vi "FGV Automatic start.vi"(11 "error in (no error)":errorcluster caption="Fehler (Eingang, kein Fehler)", 13 "Aktion":T1) -> (4 "Starten":bool, 8 "AK Start":bool, 15 "error out":errorcluster caption="Fehler (Ausgang)")   [LabVIEW 2020, in "EPA 1065.lvlib" / "Dichtheitstest 1065-345.lvlib"]
uses:
  Dichtheitstest 1065-345.lvlib
  Aktion FGV Automatic start.ctl
  Bildwechsel/Bild-Auswahl.ctl
  Bildwechsel/Bildwechsel.lvlib
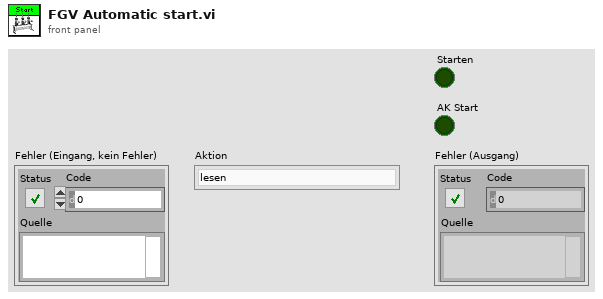
[diagram p1: front panel]
types:
  T1 = typedef "EPA 1065.lvlib/Dichtheitstest 1065-345.lvlib/Aktion FGV Automatic start.ctl" = enum16{"lesen", "Test starten aktiv", "Test starten inaktiv", "Seite merken", "Seite zurücksetzen", "AK Start inaktiv"}
  T2 = typedef "Bildwechsel.lvlib/Bild-Auswahl.ctl" = enum16{"lesen", "Initialisieren", "Beenden", "Grafik", "Anlagenübersicht", "Anlagengrenzwerte", "Log Konfig", "Gaszuordnung AO", "Erw. Konfiguration", "FT-IR  ", "Störmeldungen", "Störmeldepuffer", "Störmeldekonfig", "PNS Grenzwerte", "Statusübersicht", "Linearisierung", "ARN", "EPA Dichtheitstest", "FID", "PMA", "CalGas", "Lambda", "Interference", "Amium PNS", "EPA T90", "Interference N2O", "Scheduler", "Systemeinstellungen", "EPA Drift", "CAN Konfig"}
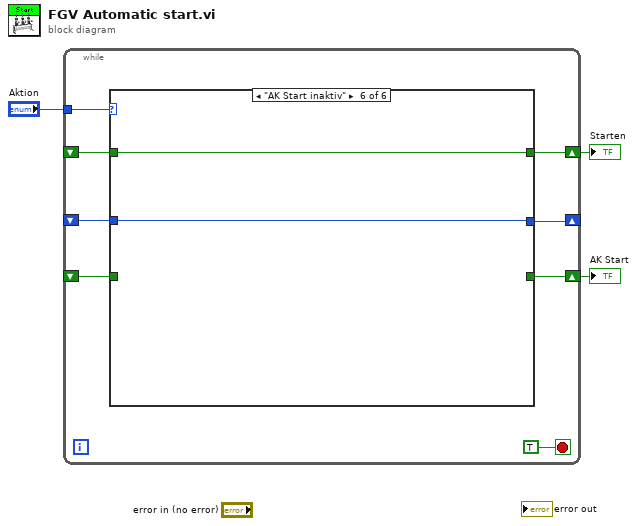
[diagram p0: block diagram]
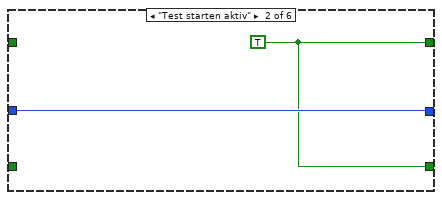
[diagram p3: hidden frame]
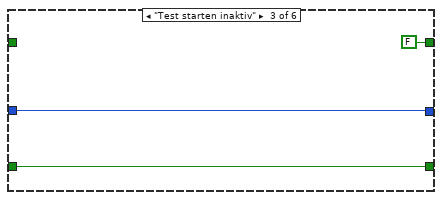
[diagram p4: hidden frame]
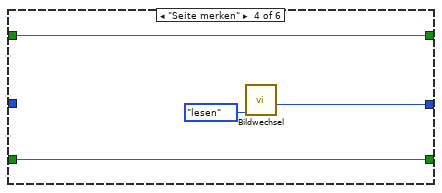
[diagram p5: hidden frame]
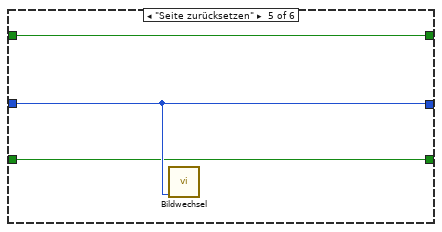
[diagram p6: hidden frame]
diagram:
  n1 = while {
    tunnel: "Aktion" -> [w10]
    shift-right: [w9] -> w2
    shift-left: _ -> [w8]
    shift-right: [w7] -> _
    shift-left: _ -> [w6]
    shift-right: [w5] -> w1
    shift-left: _ -> [w4]
    stop <- TRUE stop-if-true
    n2 = case shown="\"AK Start inaktiv\"" w10 {
      tunnel: [w14 w15 FALSE w23 w26 w27] -> w9
      tunnel: w8 -> [w14 _ _ w23 w26 w27]
      tunnel: [w13 w16 w18 w21 w25 w28] -> w7
      tunnel: w6 -> [w13 w16 w18 _ w25 w28]
      tunnel: [w12 w15 w17 w20 w24 _] -> w5
      tunnel: w4 -> [w12 _ w17 w20 w24 _]
      frame "lesen", Default {
      }
      frame "Test starten aktiv" {
        w15 = TRUE
      }
      frame "Test starten inaktiv" {
      }
      frame "Seite merken" {
        n3 = call "Bildwechsel.vi"("nächstes Bild"=Bild-Auswahl."lesen") -> ("aktuelle Bildnummer"=w21:T2)  [unwired: 9 in, 1 out]
      }
      frame "Seite zurücksetzen" {
        n4 = call "Bildwechsel.vi"("nächstes Bild"=w25) -> ()  [unwired: 9 in, 2 out]
      }
      frame "AK Start inaktiv" {
      }
    }
  }
  "Starten" <- w2
  "AK Start" <- w1
